vi "轴&IO配置检测.vi"(8 "错误输入（无错误）":errorcluster, 11 "配置检索操作":T4) -> (0 "error out":errorcluster, 2 "输出配置提取集合":T3, 3 "输入配置提取集合":T3)   [LabVIEW 2017]
panel:
  in  "输入":T1
  in  "输出":T2
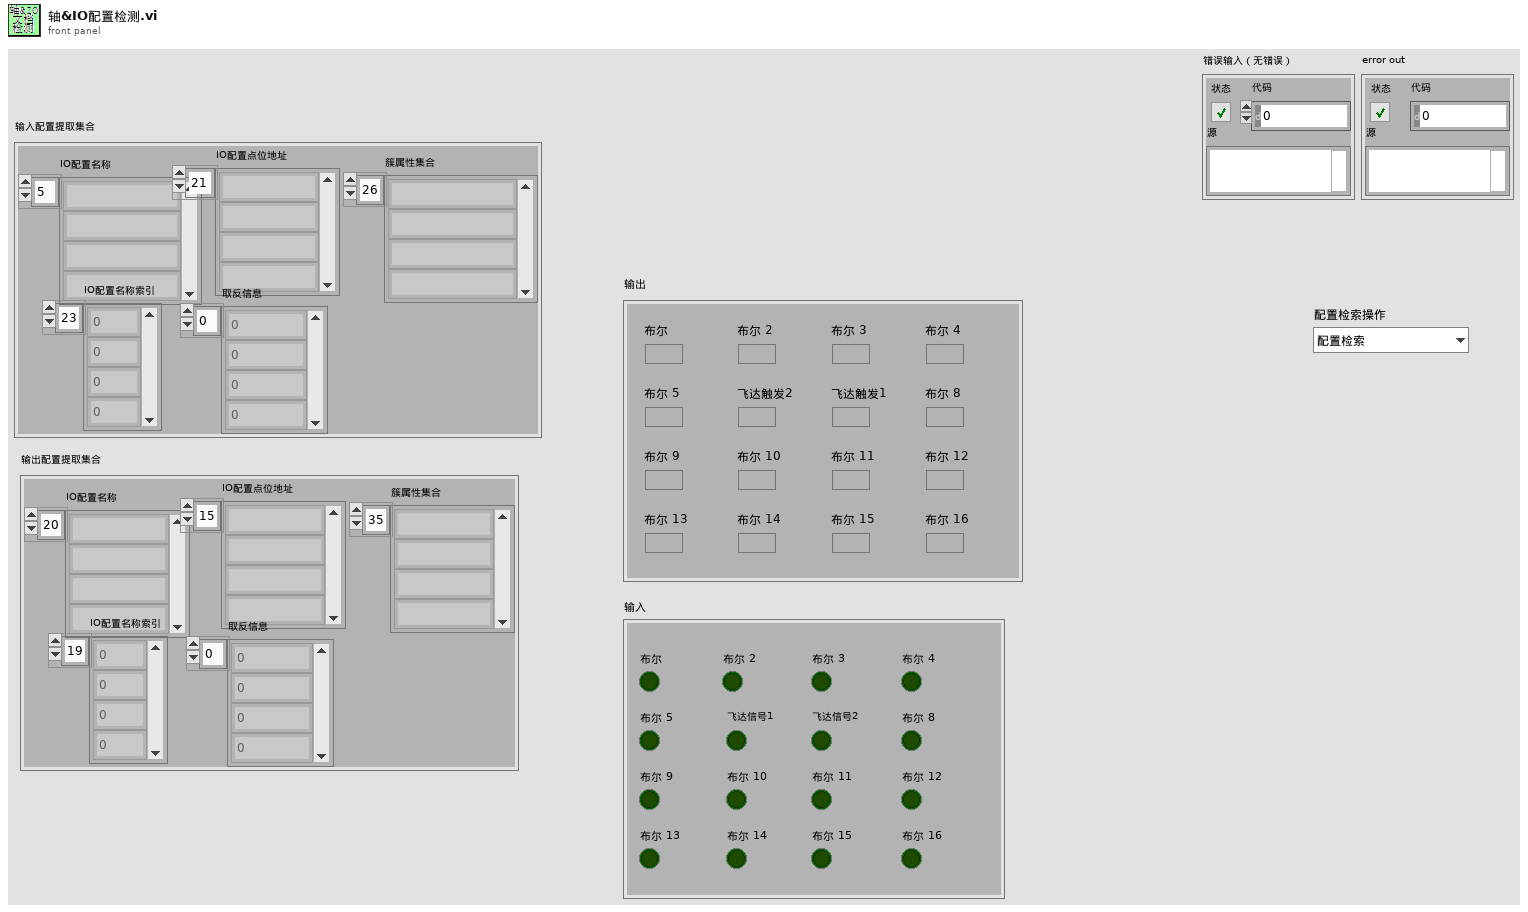
[diagram p1: front panel]
types:
  T1 = typedef "input控件.ctl" = cluster{"布尔":bool, "布尔 2":bool, "布尔 3":bool, "布尔 4":bool, "布尔 5":bool, "飞达信号1":bool, "飞达信号2":bool, "布尔 8":bool, "布尔 9":bool, "布尔 10":bool, "布尔 11":bool, "布尔 12":bool, "布尔 13":bool, "布尔 14":bool, "布尔 15":bool, "布尔 16":bool}
  T2 = typedef "output控件.ctl" = cluster{"布尔":bool, "布尔 2":bool, "布尔 3":bool, "布尔 4":bool, "布尔 5":bool, "飞达触发2":bool, "飞达触发1":bool, "布尔 8":bool, "布尔 9":bool, "布尔 10":bool, "布尔 11":bool, "布尔 12":bool, "布尔 13":bool, "布尔 14":bool, "布尔 15":bool, "布尔 16":bool}
  T3 = typedef "输入&输出配置提取集合.ctl" = cluster{"IO配置名称":string[], "IO配置点位地址":string[], "IO配置名称索引":i32[], "取反信息":i32[], "簇属性集合":string[]}
  T4 = typedef "配置检索操作.ctl" = enum16{"配置检索", "名称提取", "寄存器提取"}
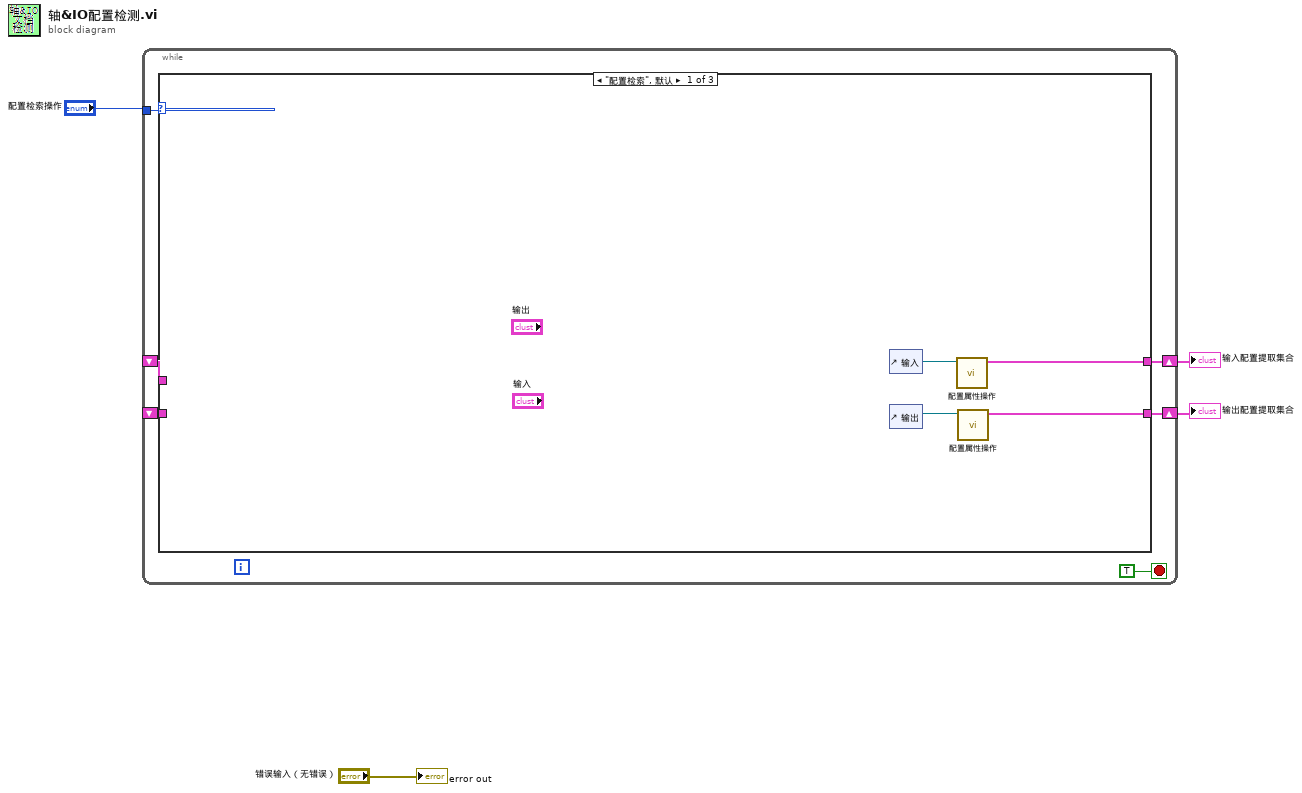
[diagram p0: block diagram]
diagram:
  n1 = while {
    tunnel: "配置检索操作" -> [w9]
    shift-right: [w8] -> w2
    shift-left: _ -> [w6]
    shift-right: [w7] -> w1
    shift-left: _ -> [w5]
    stop <- TRUE stop-if-true
    n2 = case shown="\"配置检索\", 默认" w9 {
      tunnel: [w14 w16 w18] -> w8
      tunnel: [w13 w15 w17] -> w7
      tunnel: w6 -> [_ w16 w18]
      tunnel: w5 -> [_ w15 w17]
      frame "配置检索", Default {
        n3 = control-ref of="输入"() -> (w11:refnum<vi>)
        n4 = control-ref of="输出"() -> (w12:refnum<vi>)
        n5 = call "配置属性操作.vi"("引用"=w11) -> ("配置提取集合"=w14:T3)  [unwired: 7 in, 1 out]
        n6 = call "配置属性操作.vi"("引用"=w12) -> ("配置提取集合"=w13:T3)  [unwired: 7 in, 1 out]
      }
      frame "名称提取" {
      }
      frame "寄存器提取" {
      }
    }
  }
  "输入配置提取集合" <- w2
  "输出配置提取集合" <- w1
  "error out" <- "错误输入（无错误）"
